vi "认识条件结构.vi"() -> ()   [LabVIEW 2018]
panel:
  out "字符串":string="条件结构的应用"
  in  "停止":bool
  in  "组合框":string(combo)
  out "绿色":bool
  out "黄色":bool
  out "红色":bool
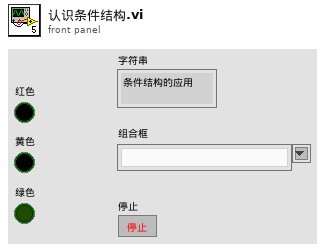
[diagram p1: front panel]
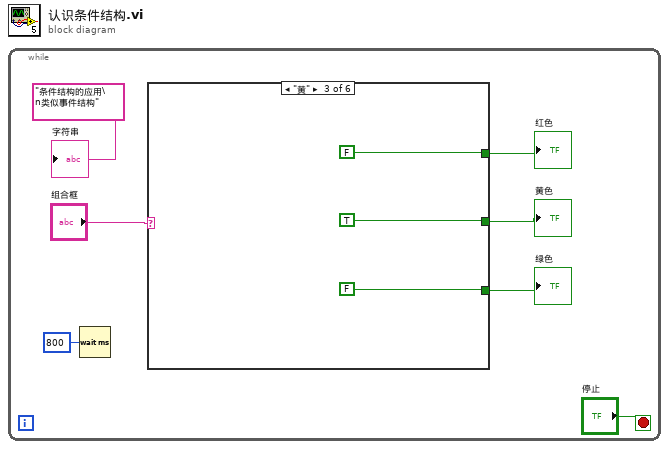
[diagram p0: block diagram]
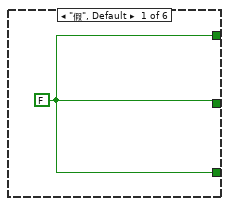
[diagram p2: hidden frame]
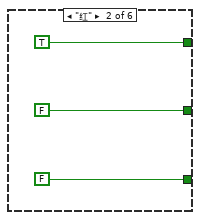
[diagram p3: hidden frame]
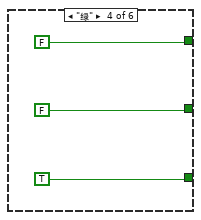
[diagram p4: hidden frame]
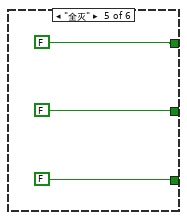
[diagram p5: hidden frame]
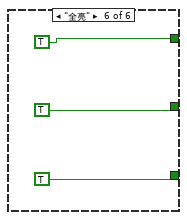
[diagram p6: hidden frame]
diagram:
  n1 = while {
    stop <- "停止" stop-if-true
    n2 = Wait (ms)(milliseconds to wait=u32 800 ("等待时间（毫秒）")) -> ()  [unwired: 1 out]
    n3 = case shown="\"黄\"" "组合框" {
      tunnel: [w8 TRUE FALSE FALSE FALSE TRUE] -> w6
      tunnel: [w8 FALSE TRUE FALSE FALSE TRUE] -> w5
      tunnel: [w8 FALSE FALSE TRUE FALSE TRUE] -> w4
      frame "假", Default {
        w8 = FALSE
      }
      frame "红" {
      }
      frame "黄" {
      }
      frame "绿" {
      }
      frame "全灭" {
      }
      frame "全亮" {
      }
    }
    "红色" <- w6
    "黄色" <- w5
    "绿色" <- w4
    "字符串" <- "条件结构的应用\n类似事件结构"
  }
